vi "Read SIMULATED_ NXP.vi"(8 "error in (no error)":errorcluster, 11 "NXP in":refnum<class "NXP.lvclass">) -> (0 "error out":errorcluster, 2 "SIMULATED?":bool, 3 "NXP out":refnum<class "NXP.lvclass">)   [LabVIEW 2019, in "NXP.lvclass"]
uses:
  NXP.lvclass
  NXP.lvclass/NXP.ctl
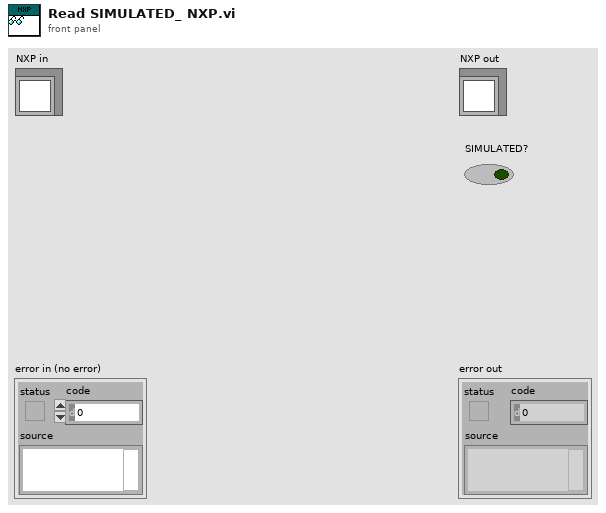
[diagram p1: front panel]
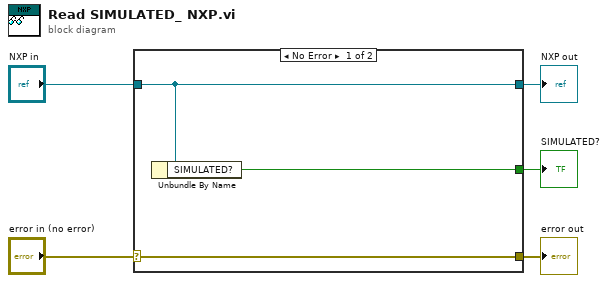
[diagram p0: block diagram]
diagram:
  n1 = case shown="No Error" "error in (no error)" {
    selector: "error in (no error)" -> [w8 w9]
    tunnel: [w8 w9] -> w4
    tunnel: [w7 w10] -> w2
    tunnel: "NXP in" -> [w7 w10]
    tunnel: [w6 _] -> w1
    frame No Error {
      n2 = Unbundle By Name(w7) -> ("SIMULATED?"=w6:bool)
    }
    frame Error {
    }
  }
  "error out" <- w4
  "NXP out" <- w2
  "SIMULATED?" <- w1
